vi "saveShopInfo.vi"(0 "数组":cluster{"ID":dbl, "食品名称":string, "价格":dbl}[](array[cluster])) -> ()   [LabVIEW 2013, in "ShopBase.lvclass"]
uses:
  ShopBase.lvclass
  <vilib>/Utility/xml.llb/Write to XML File(string).vi
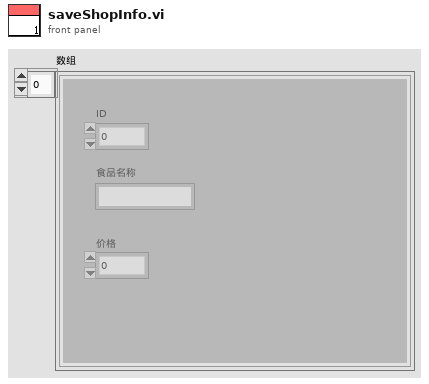
[diagram p1: front panel]
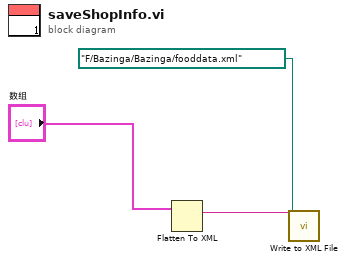
[diagram p0: block diagram]
diagram:
  n1 = Flatten To XML(anything="数组") -> (xml string=w2:string)
  n2 = call-poly <vilib>:"Write to XML File.vi"("XML Input"=w2, "XML File Path"=path "F:/Bazinga/Bazinga/fooddata.xml") -> ()  [unwired: 7 in, 3 out]
